vi "Expand Obsticle Size.vi"(1 "Map In":dbl[][](array[numeric])) -> (0 "Map Out":dbl[][](array[numeric]))   [LabVIEW 2012]
uses:
  <vilib>/Analysis/2dsp.llb/2D Convolution (DBL).vi
  <vilib>/Analysis/NI_AALPro.lvlib
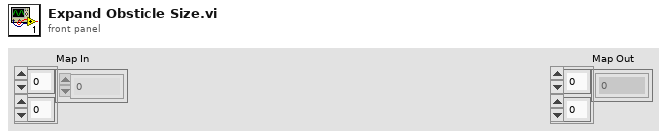
[diagram p1: front panel]
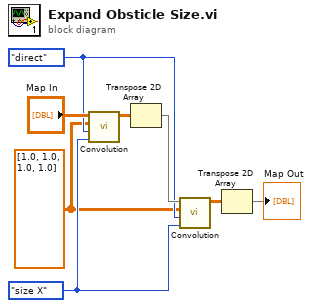
[diagram p0: block diagram]
diagram:
  w4 = enum32{"full", "size X", "compact"}."size X" ("output size")
  w3 = dbl[][] [[1.0], [1.0], [1.0], [1.0]] ("Y")
  w5 = enum32{"direct", "frequency domain"}."direct" ("algorithm")
  n1 = call-poly <vilib>:"Convolution.vi"("output size"=w4, "algorithm"=w5, "Y"=w3, "X"="Map In") -> ("X * Y"=w6:dbl[][])  [unwired: 6 in, 1 out]
  n2 = Transpose 2D Array(2D array=w6) -> (transposed array=w7:dbl[][])
  n3 = call-poly <vilib>:"Convolution.vi"("output size"=w4, "algorithm"=w5, "Y"=w3, "X"=w7) -> ("X * Y"=w2:dbl[][])  [unwired: 6 in, 1 out]
  n4 = Transpose 2D Array(2D array=w2) -> (transposed array=→"Map Out":dbl[][])
